vi "util-address-builder.vi"(9 "Channel":u8 format="%02d", 10 "Device":u8 format="%02d") -> (2 "ADDR":T1 format="%04d")   [LabVIEW 2024]
uses:
  controls/type.address.ctl
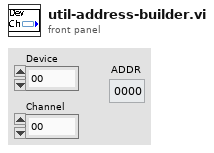
[diagram p1: front panel]
types:
  T1 = typedef "type.address.ctl" = u16
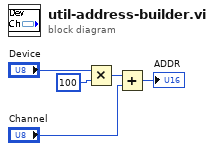
[diagram p0: block diagram]
diagram:
  n1 = Multiply(x="Device", y=u16 100) -> (x*y=w4:u16)
  n2 = Add(x=w4, y="Channel") -> (x+y=→"ADDR":u16)
